vi "log_file_setup.vi"(11 "dev-mode":bool) -> (0 "error out":errorcluster, 2 "error?":bool, 3 "appended path":path)   [LabVIEW 2024]
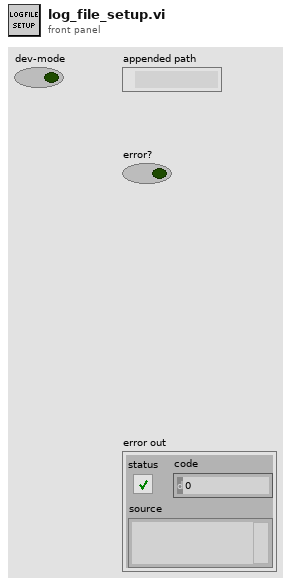
[diagram p1: front panel]
types:
  T1 = enum16{"open", "replace", "create", "open or create", "replace or create", "replace or create with confirmation"}
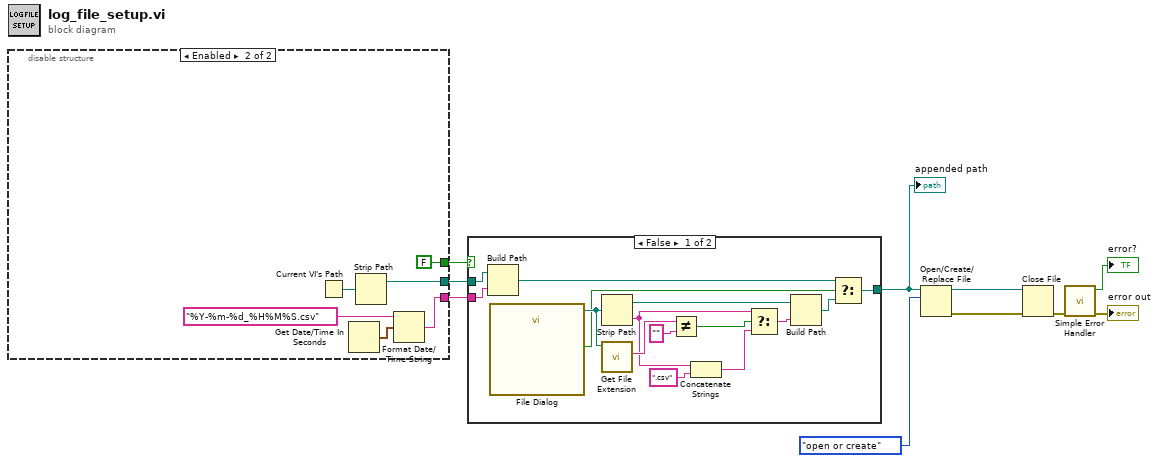
[diagram p0: block diagram]
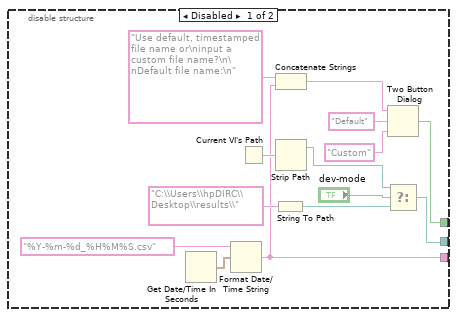
[diagram p2: hidden frame]
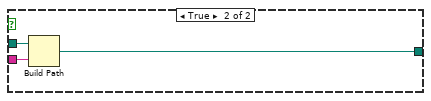
[diagram p3: hidden frame]
diagram:
  n1 = disable-structure shown="Enabled" {
    disable-tunnel: [w21 w29] -> w10
    disable-tunnel: [w18 w25] -> w4
    disable-tunnel: [w17 FALSE ("T button?")] -> w3
    frame Disabled {
      n2 = Get Date/Time In Seconds() -> (seconds since 1Jan1904=w11:timestamp)
      n3 = Format Date/Time String(time format string (%c)="%Y-%m-%d_%H%M%S.csv", seconds (now)=w11) -> (date/time string=w18:string)  [unwired: 1 in]
      n4 = Current VI's Path() -> (path=w19:path)
      n5 = String To Path(string="C:\\Users\\hpDIRC\\Desktop\\results\\" ("T button name (\"OK\")")) -> (path=w22:path)
      n6 = Concatenate Strings("Use default, timestamped file name or\ninput a custom file name?\n\nDefault file name:\n", w18) -> (w14:string)
      n7 = Strip Path(path=w19) -> (stripped path=w23:path)  [unwired: 1 out]
      n8 = Two Button Dialog(message=w14, 1:"Custom" ("T button name (\"OK\")"), 2:"Default" ("T button name (\"OK\")")) -> (T button?=w17:bool)
      n9 = Select(t=w23, s="dev-mode", f=w22) -> (s? t:f=w21:path)
    }
    frame Enabled {
      n10 = Current VI's Path() -> (path=w30:path)
      n11 = Get Date/Time In Seconds() -> (seconds since 1Jan1904=w27:timestamp)
      n12 = Strip Path(path=w30) -> (stripped path=w29:path)  [unwired: 1 out]
      n13 = Format Date/Time String(time format string (%c)="%Y-%m-%d_%H%M%S.csv", seconds (now)=w27) -> (date/time string=w25:string)  [unwired: 1 in]
    }
  }
  n14 = case shown="False" w3 {
    tunnel: w4 -> [w35 w48]
    tunnel: [w32 w47] -> w6
    tunnel: w10 -> [w31 w46]
    frame False {
      n15 = Build Path(base path=w31, name or relative path=w35) -> (appended path=w34:path)
      n16 = call "File Dialog"() -> ("selected path"=w38:path, "cancelled"=w36:bool)  [unwired: 12 in, 2 out]
      n17 = Strip Path(path=w38) -> (stripped path=w39:path, name=w40:string)
      n18 = call <vilib>:"Get File Extension.vi"("file"=w38) -> ("lowercase file extension"=w45:string)  [unwired: 6 in, 4 out]
      n19 = Not Equal?(x=w45, y="") -> (x != y?=w42:bool)
      n20 = Concatenate Strings(w40, ".csv" ("string")) -> (w41:string)
      n21 = Select(t=w40, s=w42, f=w41) -> (s? t:f=w37:string)
      n22 = Build Path(base path=w39, name or relative path=w37) -> (appended path=w33:path)
      n23 = Select(t=w34, s=w36, f=w33) -> (s? t:f=w32:path)
    }
    frame True {
      n24 = Build Path(base path=w46, name or relative path=w48) -> (appended path=w47:path)
    }
  }
  "appended path" <- w6
  n25 = Open/Create/Replace File(file path (use dialog)=w6, operation (0:open)=T1."open or create") -> (refnum out=w2:refnum<file>, error out=w1:errorcluster)  [unwired: 4 in, 1 out]
  n26 = Close File(refnum=w2, error in=w1) -> (error out=w7:errorcluster)  [unwired: 1 out]
  n27 = call <vilib>:"Simple Error Handler.vi"("error in (no error)"=w7) -> ("error?"=→"error?":bool, "error out"=→"error out":errorcluster)  [unwired: 4 in, 3 out]
